vi "BRig_RT__Case_Exp__State_start__sendExpData_uploadData__v2.vi"(9 "input_error":errorcluster, 10 "input_hSession":T1, 11 "input_connected":bool) -> (3 "output_sent":bool)   [LabVIEW 2014]
uses:
  <vilib>/WebDAVClient/Advanced/SessionHandle.ctl
  <vilib>/WebDAVClient/Advanced/Put File.vi
  <vilib>/WebDAVClient/NI_WebDAV.lvlib
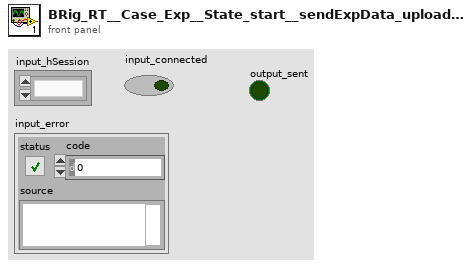
[diagram p1: front panel]
types:
  T1 = typedef "NI_WebDAV.lvlib/SessionHandle.ctl" = refnum<k1>
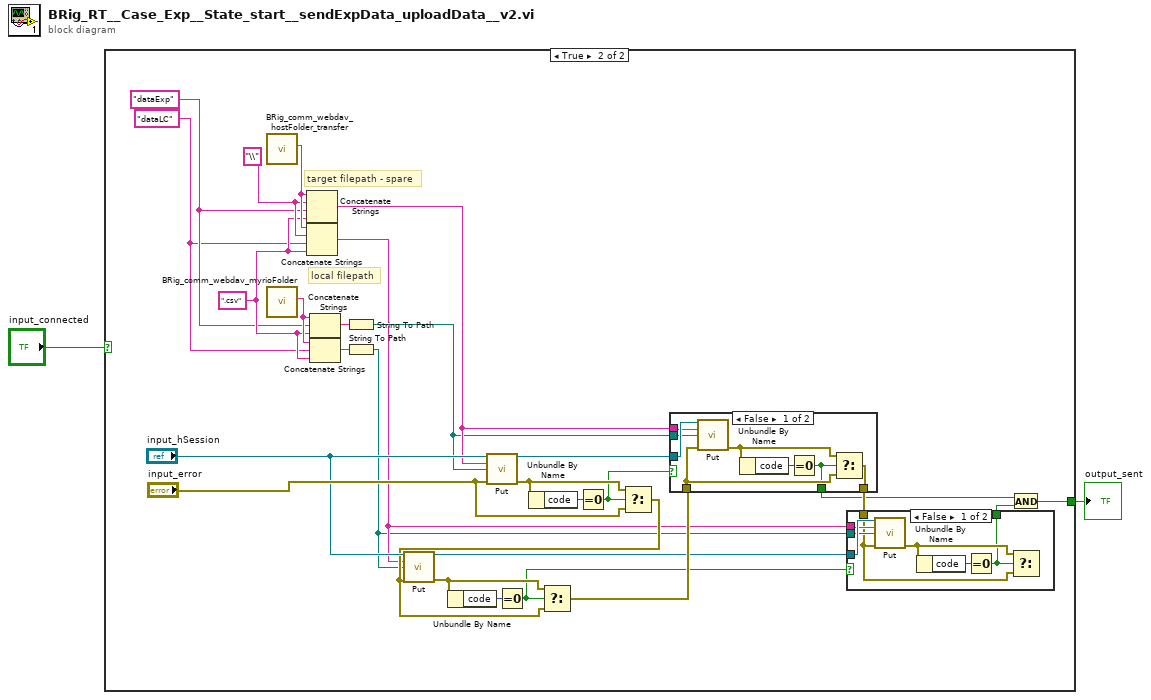
[diagram p0: block diagram]
diagram:
  n1 = case shown="True" "input_connected" {
    tunnel: [_ w3] -> w1
    frame False {
    }
    frame True {
      w26 = "\\" ("string")
      w23 = "dataLC" ("input_filename")
      w24 = "dataExp" ("input_filename")
      w25 = ".csv" ("string")
      # "target filepath - spare"
      # "local filepath"
      n2 = call "BRig_comm_webdav_hostFolder_transfer.vi"() -> ("output_HostFolder"=w27:string)  [unwired: 11 in]
      n3 = call "BRig_comm_webdav_myrioFolder.vi"() -> ("output_myrioFolder"=w28:string)  [unwired: 11 in]
      n4 = Concatenate Strings(w27, w26, w24, w25) -> (w12:string)
      n5 = Concatenate Strings(w27, w26, w23, w25) -> (w9:string)
      n6 = Concatenate Strings(w28, w24, w25) -> (w30:string)
      n7 = Concatenate Strings(w28, w23, w25) -> (w29:string)
      n8 = String To Path(string=w30) -> (path=w11:path)
      n9 = String To Path(string=w29) -> (path=w8:path)
      n10 = call-poly <vilib>:"Put.vi"("session handle"="input_hSession", "relative uri"=w12, "local file path"=w11, "error in (no error)"="input_error") -> ("session handle out"=w13:T1, "error out"=w21:errorcluster)  [unwired: 9 in, 1 out]
      n11 = Unbundle By Name(w21) -> ("code"=w22:i32)
      n12 = Equal To 0?(x=w22) -> (x = 0?=w15:bool)
      n13 = Select(t=w21, s=w15, f="input_error") -> (s? t:f=w16:errorcluster)
      n14 = call-poly <vilib>:"Put.vi"("session handle"="input_hSession", "relative uri"=w9, "local file path"=w8, "error in (no error)"=w16) -> ("session handle out"=w10:T1, "error out"=w17:errorcluster)  [unwired: 9 in, 1 out]
      n15 = Unbundle By Name(w17) -> ("code"=w18:i32)
      n16 = Equal To 0?(x=w18) -> (x = 0?=w7:bool)
      n17 = Select(t=w17, s=w7, f=w16) -> (s? t:f=w14:errorcluster)
      n18 = case shown="False" w15 {
        selector: w15 -> [_ w47]
        tunnel: w14 -> [w44 w48]
        tunnel: w13 -> [w43 _]
        tunnel: w12 -> [w42 _]
        tunnel: w11 -> [w41 _]
        tunnel: [w40 w48] -> w6
        tunnel: [w39 w47] -> w5
        frame False {
          n19 = call-poly <vilib>:"Put.vi"("session handle"=w43, "relative uri"=w42, "local file path"=w41, "error in (no error)"=w44) -> ("error out"=w46:errorcluster)  [unwired: 9 in, 2 out]
          n20 = Unbundle By Name(w46) -> ("code"=w45:i32)
          n21 = Equal To 0?(x=w45) -> (x = 0?=w39:bool)
          n22 = Select(t=w46, s=w39, f=w44) -> (s? t:f=w40:errorcluster)
        }
        frame True {
        }
      }
      n23 = case shown="False" w7 {
        selector: w7 -> [_ w38]
        tunnel: w10 -> [w35 _]
        tunnel: w9 -> [w34 _]
        tunnel: w8 -> [w33 _]
        tunnel: w6 -> [w32 _]
        tunnel: [w31 w38] -> w4
        frame False {
          n24 = call-poly <vilib>:"Put.vi"("session handle"=w35, "relative uri"=w34, "local file path"=w33, "error in (no error)"=w32) -> ("error out"=w37:errorcluster)  [unwired: 9 in, 2 out]
          n25 = Unbundle By Name(w37) -> ("code"=w36:i32)
          n26 = Equal To 0?(x=w36) -> (x = 0?=w31:bool)
          n27 = Select(t=w37, s=w31, f=w32) -> ()  [unwired: 1 out]
        }
        frame True {
        }
      }
      n28 = And(x=w5, y=w4) -> (x .and. y?=w3:bool)
    }
  }
  "output_sent" <- w1
